vi "Send MsgQ.vi"(8 "error in (no error)":errorcluster, 9 "Data In":variant, 10 "Message String":string, 11 "Send to MsgQ":T1) -> (0 "error out":errorcluster)   [LabVIEW 2013, in "Main MsgQ.lvlib"]
uses:
  Main MsgQ.lvlib
  MsgQ Loops enum.ctl
  Common/Interloop MessageQ/Message que instance modes enum.ctl
  Common/Interloop MessageQ/Interloop MessageQ.lvlib
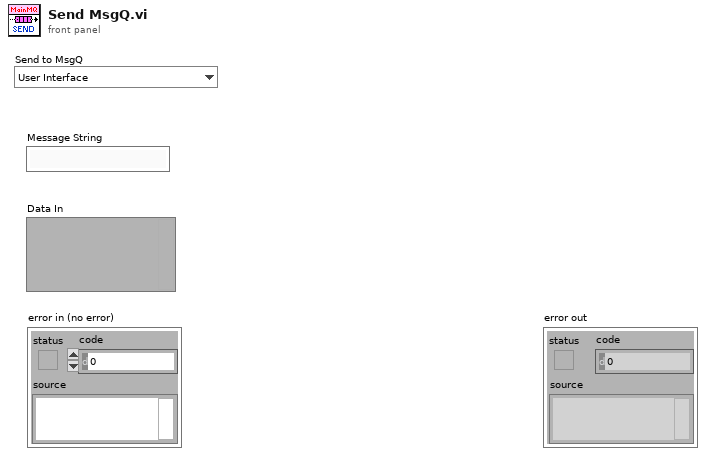
[diagram p1: front panel]
types:
  T1 = typedef "Main MsgQ.lvlib/MsgQ Loops enum.ctl" = enum16{"User Interface", "Image Acq"}
  T2 = typedef "Interloop MessageQ.lvlib/Message que instance modes enum.ctl" = enum16{"Initialize", "Broadcast Message", "Send Message", "Read Message", "Kill"}
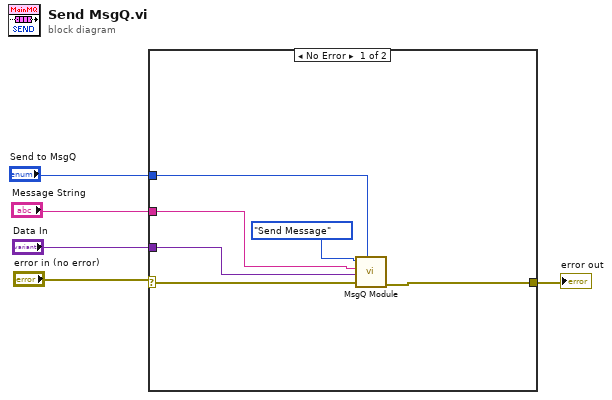
[diagram p0: block diagram]
diagram:
  n1 = case shown="No Error" "error in (no error)" {
    selector: "error in (no error)" -> [w8 w12]
    tunnel: [w7 w12] -> w4
    tunnel: "Send to MsgQ" -> [w6 _]
    tunnel: "Message String" -> [w10 _]
    tunnel: "Data In" -> [w9 _]
    frame No Error {
      n2 = call "MsgQ Module.vi"("MsgQ enum"=w6, "error in (no error)"=w8, "Message Send Parameters"=w9, "Message Send String"=w10, "Mode"=Message_que_instance_modes_enum."Send Message") -> ("error out"=w7:errorcluster)  [unwired: 3 in, 3 out]
    }
    frame Error {
    }
  }
  "error out" <- w4
